vi "Induction Range.vi"(8 "Error In":errorcluster) -> (0 "Error Out":errorcluster)   [LabVIEW 2016]
uses:
  Utility/LabVIEW GEA2 Toolkit v1.0.0.0/type defs/ERD Read Data In.ctl
  Utility/LabVIEW GEA2 Toolkit v1.0.0.0/type defs/Data Type.ctl
  Utility/LabVIEW GEA2 Toolkit v1.0.0.0/type defs/Source_Destination.ctl
  Utility/LabVIEW GEA2 Toolkit v1.0.0.0/library/GEA2_Toolkit.lvlib
panel:
  in  "Tab Control":enum32{"Main", "Debug"}(tab)
  out "Data":string[][](array[string])
  in  "Scan Rate (sec)":u32=1
  in  "Read ERD List":T1[](array[typedef])=[{"ERD Number"=62219, "Data Type"=enum."uint16_t"}, {"ERD Number"=62246, "Data Type"=enum."uint32_t"}, {"ERD Number"=62247, "Data Type"=enum."uint32_t"}, {"ERD Number"=62723, "Data Type"=enum."uint16_t"}, {"ERD Number"=62724, "Data Type"=enum."uint16_t"}] {"ERD Number" format="%.0x"}
  in  "stop":bool
  in  "Choose Folder":path
  in  "Save Data":bool
  in  "Board Index (Green Bean 0-3)":i32
  in  "GEA Inputs":T3={"Source"=228, "Destination"=136} {"Destination" format="%.0x"; "Source" format="%.0x"}
  in  "#ERDs per message":i32=5
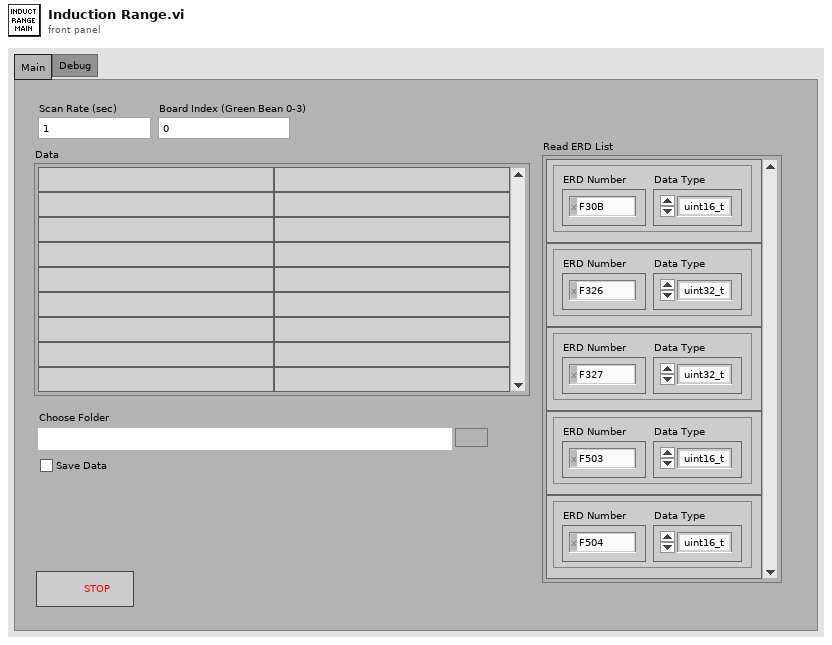
[diagram p1: front panel]
types:
  T1 = typedef "GEA2_Toolkit.lvlib/ERD Read Data In.ctl" = cluster{"ERD Number":u16, "Data Type":T2}
  T2 = typedef "GEA2_Toolkit.lvlib/Data Type.ctl" = enum16{"string", "boolean", "uint8_t", "uint16_t", "uint32_t", "uint64_t"}
  T3 = typedef "GEA2_Toolkit.lvlib/Source_Destination.ctl" = cluster{"Source":u8, "Destination":u8}
  T4 = typedef "GEA2_Toolkit.lvlib/ERD Read Data Out.ctl" = cluster{"ERD Number":u16, "Data":string}
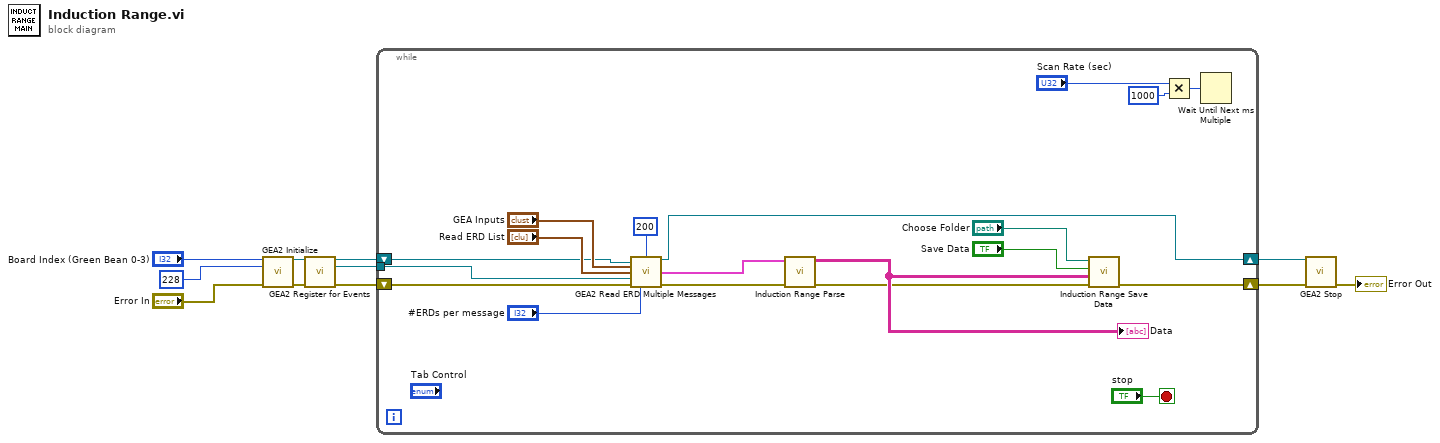
[diagram p0: block diagram]
diagram:
  n1 = call "GEA2 Initialize.vi"("Board Index"="Board Index (Green Bean 0-3)", "Source Address"=u8 228, "error in"="Error In") -> ("GEA2 Reference Out"=w11:refnum<k24>, "error out"=w10:errorcluster)  [unwired: 10 in, 1 out]
  n2 = call "GEA2 Register for Events.vi"("GEA2 Reference In"=w11, "Error In"=w10) -> ("GEA2 Reference Out"=w6:refnum<k24>, "GEA2 Event Registration"=w5:refnum<event-registration>, "Error Out"=w7:errorcluster)  [unwired: 11 in]
  n3 = while {
    tunnel: w5 -> [w24]
    shift-right: [w12] -> w4
    shift-left: w7 -> [w26]
    shift-right: [w23] -> w3
    shift-left: w6 -> [w25]
    stop <- "stop" stop-if-true
    n4 = call "GEA2 Read ERD Multiple Messages.vi"("GEA2 Reference In"=w25, "Read Timeout (ms)"=u32 200, "GEA Inputs"="GEA Inputs", "Read ERD List"="Read ERD List", "GEA2 Event Registration"=w24, "Error In"=w26, "#ERDs per message"="#ERDs per message") -> ("GEA2 Reference Out"=w23:refnum<k24>, "ERD Data Out"=w21:T4[], "Error Out"=w20:errorcluster)  [unwired: 4 in, 2 out]
    n5 = call "Induction Range Parse.vi"("Error In"=w20, "ERD Data Out"=w21) -> ("Error Out"=w13:errorcluster, "Data"=w14:string[][])  [unwired: 8 in]
    "Data" <- w14
    n6 = call "Induction Range Save Data.vi"("Error In"=w13, "Data"=w14, "Save Data"="Save Data", "Choose Folder"="Choose Folder") -> ("Error Out"=w12:errorcluster)  [unwired: 7 in]
    n7 = Multiply(x="Scan Rate (sec)", y=u32 1000) -> (x*y=w17:u32)
    n8 = Wait Until Next ms Multiple(millisecond multiple=w17) -> ()  [unwired: 1 out]
  }
  n9 = call "GEA2 Stop.vi"("GEA2 Reference Out"=w3, "Error In"=w4) -> ("Error Out"=→"Error Out":errorcluster)  [unwired: 13 in]
